vi "Perform Action.vi"(8 "Error In":errorcluster, 10 "Input":variant, 11 "reference in":refnum<class "Instrument.lvclass">) -> (0 "Error Out":errorcluster, 2 "Output":variant, 3 "reference out":refnum<class "Instrument.lvclass">)   [LabVIEW 2023, in "HAL GOOP4.lvlib" / "Instrument.lvclass"]
uses:
  Instrument.lvclass
  Interfaces/IConfigure/IConfigure.lvclass
  Instrument.lvclass/Instrument.ctl
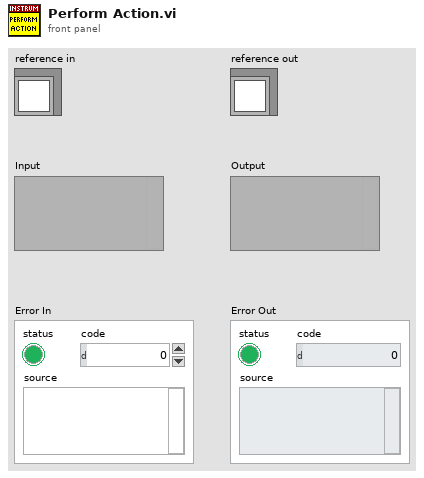
[diagram p1: front panel]
types:
  T1 = typedef "HAL GOOP4.lvlib/Instrument.lvclass/ObjectAttributes.ctl" = cluster{"IConfigure":refnum<class "IConfigure.lvclass">, "Ref Count":u8, "Start Count":u8}
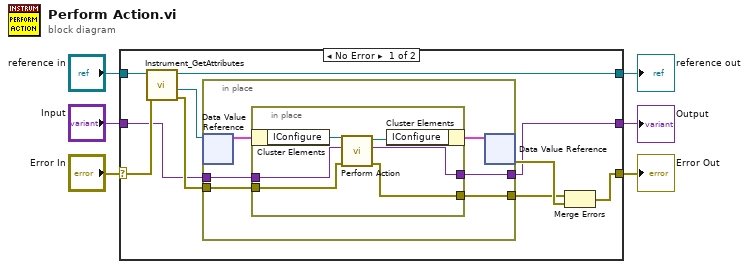
[diagram p0: block diagram]
diagram:
  n1 = case shown="No Error" "Error In" {
    selector: "Error In" -> [w16 w31]
    tunnel: [w8 w31] -> w5
    tunnel: [w14 w30] -> w3
    tunnel: "reference in" -> [w15 w30]
    tunnel: "Input" -> [w10 w29]
    tunnel: [w7 w29] -> w1
    frame No Error {
      n2 = call "Instrument_GetAttributes.vi"("Error In"=w16, "reference in"=w15) -> ("Error Out"=w11:errorcluster, "DataRef"=w12:refnum<data-value>, "reference out"=w14:refnum<class "Instrument.lvclass">)  [unwired: 6 in, 1 out]
      n3 = in-place {
        in-place-border: w11 -> [w20]
        in-place-border: w10 -> [w19]
        in-place-border: [w18] -> w7
        in-place-border: [w17] -> w9
        n4 = in-place-dvr #1(w12) -> (w22:T1)  [unwired: 1 out]
        n5 = in-place {
          in-place-border: w20 -> [w23]
          in-place-border: w19 -> [w26]
          in-place-border: [w25] -> w18
          in-place-border: [w24] -> w17
          n6 = in-place-cluster #2(w22) -> ("IConfigure"=w28:refnum<class "IConfigure.lvclass">)
          n7 = call-dynamic "Perform Action.vi"("error in (no error)"=w23, "Input"=w26, "IConfigure in"=w28) -> ("error out"=w24:errorcluster, "Output"=w25:variant, "IConfigure out"=w27:refnum<class "IConfigure.lvclass">)  [unwired: 6 in]
          n8 = in-place-cluster #2("IConfigure"=w27) -> (w21:T1)
        }
        n9 = in-place-dvr #1(w21) -> (w13:errorcluster)  [unwired: 1 out]
      }
      n10 = Merge Errors(w9, w13) -> (w8:errorcluster)
    }
    frame Error {
    }
  }
  "Error Out" <- w5
  "reference out" <- w3
  "Output" <- w1
